vi "KG remote.vi"(8 "Fehler (Eingang, kein Fehler)":errorcluster, 11 "VISA-Ressourcenname":refnum<visa-resource-name>) -> (0 "Fehler (Ausgang)":errorcluster, 3 "VISA-Ressourcenname (Ausgang)":refnum<visa-resource-name>)   [LabVIEW 2020, in "Linearisierung v2.lvlib" / "Gasteiler.lvlib" / "HovaCAL_Interface.lvlib" / "KGN.lvlib" / "set.lvlib"]
uses:
  set.lvlib
  KGN.lvlib
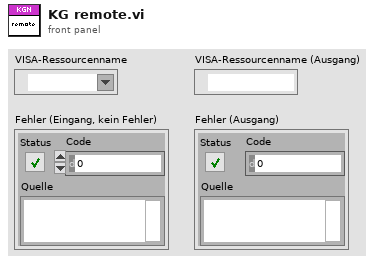
[diagram p1: front panel]
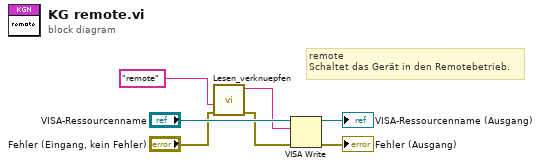
[diagram p0: block diagram]
diagram:
  # "remote\nSchaltet das Gerät in den Remotebetrieb."
  n1 = call "Lesen_verknuepfen.vi"("error in (no error)"="Fehler (Eingang, kein Fehler)", "Order"="remote" ("Schreibpuffer")) -> ("error out"=w3:errorcluster, "Verknüpfter String"=w2:string)  [unwired: 8 in]
  n2 = VISA Write(VISA resource name="VISA-Ressourcenname", write buffer=w2, error in (no error)=w3) -> (VISA resource name out=→"VISA-Ressourcenname (Ausgang)":refnum<visa-resource-name>, error out=→"Fehler (Ausgang)":errorcluster)  [unwired: 1 out]
